vi "Global_var.vi"() -> ()   [LabVIEW 2023]
panel:
  out "Reset Buffer Count":dbl
  out "Mesure":dbl
  out "Time Boucle After":dbl
  out "Time Boucle Before":dbl
  out "Durée Boucle":dbl
  out "Path Save":path
  out "Path Template":path
  out "Tension Sent (V) Z":dbl
  out "Tension Sent (V) Y":dbl
  out "Tension Sent (V) X":dbl
  out "Local Acc Z":dbl
  out "Local Acc Y":dbl
  out "Local Acc X":dbl
  out "Base Tension (V) Z":dbl
  out "Base Tension (V) Y":dbl
  out "Base Tension (V) X":dbl
  out "Base Acc Z":dbl
  out "Base Acc Y":dbl
  out "Base Acc X":dbl
  out "Mode ACT":dbl
  out "Acc Z":dbl
  out "Acc Y":dbl
  out "Acc X":dbl
  out "Speed Instant Z":dbl
  out "Speed Instant Y":dbl
  out "Speed Instant X":dbl
  out "Local Speed Z":dbl
  out "Local Speed Y":dbl
  out "Local Speed X":dbl
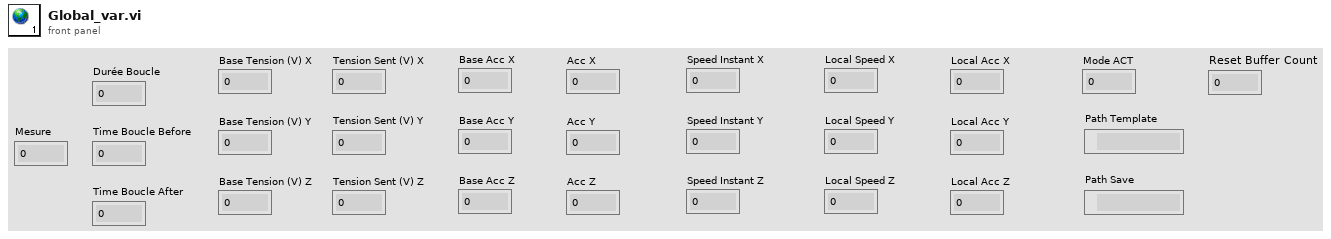
[diagram p1: front panel]
diagram:
